vi "FTW-Reflection-Cluster.vi"(7 "Cluster":variant) -> (8 "Cluster Elements":T2(array[cluster]))   [LabVIEW 2013]
uses:
  FTW-Reflection-Types.ctl
panel:
  # "Inputs"
  # "Outputs"
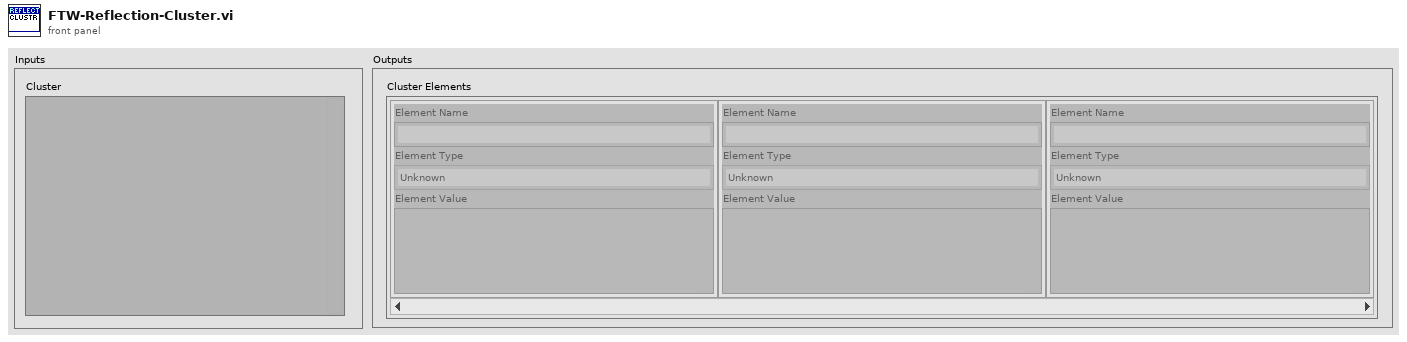
[diagram p1: front panel]
types:
  T1 = typedef "FTW-Reflection-Types.ctl" = enum16{"Unknown", "Void", "Array", "Cluster", "LVObject", "Boolean", "I8", "I16", "I32", "I64", "U8", "U16", "U32", "U64", "SGL", "DBL", "EXT", "CSG", "CDB", "CXT", "FXP", "EnumU8", "EnumU16", "EnumU32", "EnumU64", "SGLwithUnit", "DBLwithUnit", "EXTwithUnit", "CSGwithUnit", "CDBwithUnit", "CXTwithUnit", "String", "Path", "Picture", "Tag", "LVVariant", "Timestamp", "WaveformI8", "WaveformI16", "WaveformI32", "WaveformI64", "WaveformU8", "WaveformU16", "WaveformU32", "WaveformU64", "WaveformSGL", "WaveformDBL", "WaveformEXT", "WaveformCSG", "WaveformCDB", "WaveformCXT", "WaveformDigital", "WaveformUnknownType", "DigitalData", "DynamicData", "ExternalData", "FileByteStream", "TDMStream", "dotNET", "ActiveX", "VIServerReference", "VIReference", "ApplicationInstance", "Menu", "ConnectionDataSocket", "ConnectionVISA", "ConnectionBluetooth", "ConnectionIrDA", "ConnectionTCP", "ConnectionUDP", "ConnectionHTTPClient", "ConnectionFTP", "Occurrence", "Notifier", "Queue", "Rendezvous", "Semaphore", "RTFIFO", "EventPublisher", "EventRegistration", "EventCallback", "DataValueReference", "GenericClass", "GenericClassTag", "GenericClassDeepCopy", "GenericClassFlattened", "GenericClassTagFlattened", "GenericReferenceType", "WindowsRegistry", "OverloadedDatalogRef", "ReferenceUnknownType"}
  T2 = cluster{"Element Name":string, "Element Type":T1, "Element Value":variant}[]
  T3 = cluster{"Data Name":string, "LabVIEW Type":T1, "Variant Type and Value":variant}
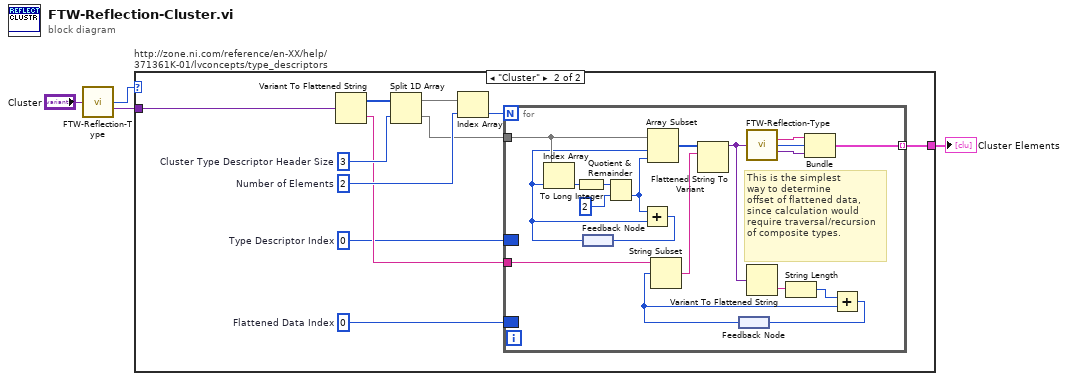
[diagram p0: block diagram]
diagram:
  n1 = call "FTW-Reflection-Type.vi"("Anything"="Cluster") -> ("LabVIEW Type"=w1:T1, "Variant Type and Value"=w2:variant)  [unwired: 12 in, 1 out]
  n2 = case "http://zone.ni.com/reference/en-XX/help/371361K-01/lvconcepts/type_descriptors" shown="\"Cluster\"" w1 {
    tunnel: [_ w13] -> w4
    tunnel: w2 -> [_ w12]
    frame Default {
    }
    frame "Cluster" {
      w8 = 0  # Flattened Data Index
      w6 = 0  # Type Descriptor Index
      w10 = 3  # Cluster Type Descriptor Header Size
      w15 = 2  # Number of Elements
      n3 = Variant To Flattened String(Variant=w12) -> (data string=w7:string, 1:w11:i16[])
      n4 = Split 1D Array(array=w11, index=w10) -> (first subarray=w5:i16[], second subarray=w9:i16[])
      n5 = Index Array(array=w5, index=w15) -> (element=w14:i16)
      n6 = for {
        N: w14 -> [_]
        tunnel: w9 -> [w30]
        tunnel: w7 -> [w26]
        tunnel: [w31] -> w13 mode=indexing
        border: w6 -> [_]
        border: w8 -> [_]
        # "This is the simplest\nway to determine\noffset of flattened data,\nsince calculation would\nrequire traversal/recursion\nof composite types."
        n7 = feedback #1() -> (w17:i32)
        n8 = Index Array(array=w30, index=w17) -> (element=w29:i16)
        n9 = To Long Integer(number=w29) -> (32bit integer=w28:i32)
        n10 = Quotient & Remainder(x=w28, y=2) -> (floor(x/y)=w27:i32)  [unwired: 1 out]
        n11 = Add(x=w27, y=w17) -> (x+y=w16:i32)
        n12 = feedback-in #1(w16) -> ()
        n13 = Array Subset(array=w30, index=w17, length=w27) -> (w21:i16[])
        n14 = feedback #2() -> (w19:i32)
        n15 = String Subset(string=w26, offset (0)=w19) -> (substring=w25:string)  [unwired: 1 in]
        n16 = Flattened String To Variant(6:w25, 7:w21) -> (3:w24:variant)  [unwired: 1 in, 1 out]
        n17 = call "FTW-Reflection-Type.vi"("Anything"=w24) -> ("Data Name"=w34:string, "LabVIEW Type"=w33:T1, "Variant Type and Value"=w32:variant)  [unwired: 12 in]
        n18 = Variant To Flattened String(Variant=w24) -> (data string=w23:string)  [unwired: 1 out]
        n19 = String Length(string=w23) -> (length=w22:i32)
        n20 = Bundle("Data Name"=w34, "LabVIEW Type"=w33, "Variant Type and Value"=w32) -> (w31:T3)  [unwired: 1 in]
        n21 = Add(x=w22, y=w19) -> (x+y=w18:i32)
        n22 = feedback-in #2(w18) -> ()
      }
    }
  }
  "Cluster Elements" <- w4
